vi "Get First Target In Sysdef.vi"(8 "error in (no error)":errorcluster, 11 "Sysdef Path":path) -> (0 "error out":errorcluster, 3 "Target":refnum<k24>)   [LabVIEW 2020, in "Engine Simulation IO System Tests.lvclass"]
uses:
  Engine Simulation IO System Tests.lvclass
  NationalInstruments.VeriStand.SystemDefinitionAPI
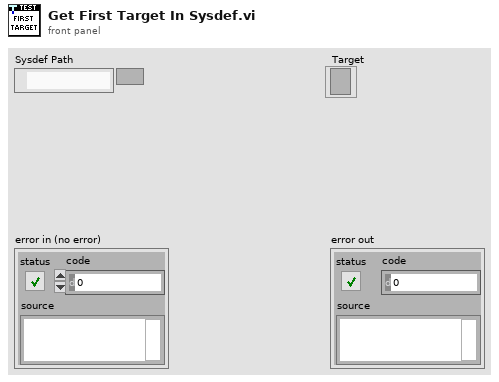
[diagram p1: front panel]
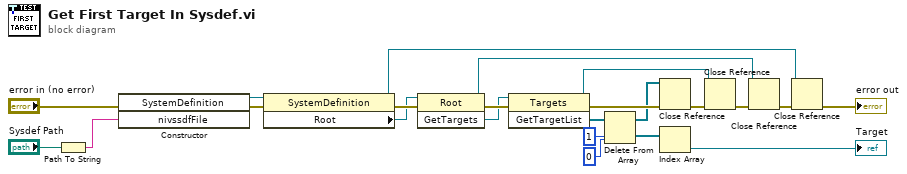
[diagram p0: block diagram]
diagram:
  n1 = Path To String(path="Sysdef Path") -> (string=w23:string)
  n2 = constructor class="SystemDefinition"(error in="error in (no error)", "nivssdfFile"=w23) -> (reference out=w9:refnum<k24>, error out=w10:errorcluster)  [unwired: 2 in, 2 out]
  n3 = property class="SystemDefinition"(reference=w9, error in=w10) -> (reference out=w5:refnum<k24>, error out=w22:errorcluster, "Root"=w21:refnum<k24>)
  n4 = invoke class="Root" method="GetTargets"(reference=w21, error in=w22) -> (reference out=w6:refnum<k24>, error out=w20:errorcluster, "GetTargets"=w19:refnum<k24>)  [unwired: 1 in]
  n5 = invoke class="Targets" method="GetTargetList"(reference=w19, error in=w20) -> (reference out=w12:refnum<k24>, error out=w15:errorcluster, "GetTargetList"=w18:refnum<k24>[])  [unwired: 1 in]
  n6 = Delete From Array(array=w18, length=1, index=0) -> (deleted portion=w11:refnum<k24>[], array with subset deleted=w14:refnum<k24>[])
  n7 = Close Reference(reference=w14, error in (no error)=w15) -> (error out=w13:errorcluster)
  n8 = Index Array(array=w11) -> (element=→"Target":refnum<k24>)  [unwired: 1 in]
  n9 = Close Reference(reference=w12, error in (no error)=w13) -> (error out=w8:errorcluster)
  n10 = Close Reference(reference=w6, error in (no error)=w8) -> (error out=w7:errorcluster)
  n11 = Close Reference(reference=w5, error in (no error)=w7) -> (error out=→"error out":errorcluster)
